vi "AguaClara license agreement.vi"(3 "year":u16) -> (0 "Accepted":bool, 1 "License":string)   [LabVIEW 2015]
panel:
  out "title":string
  in  "OK Button":bool
  in  "I do NOT accept terms of the agreement":bool=TRUE
  in  "I accept terms of the agreement":bool
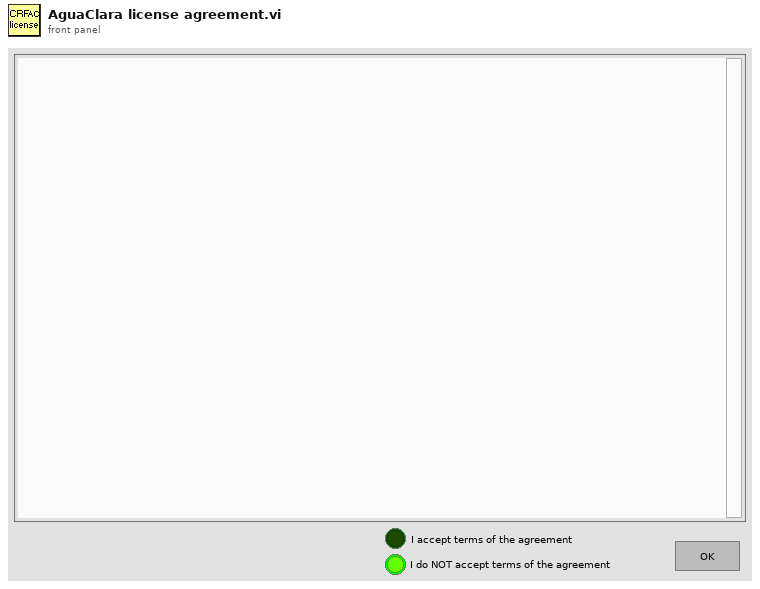
[diagram p1: front panel]
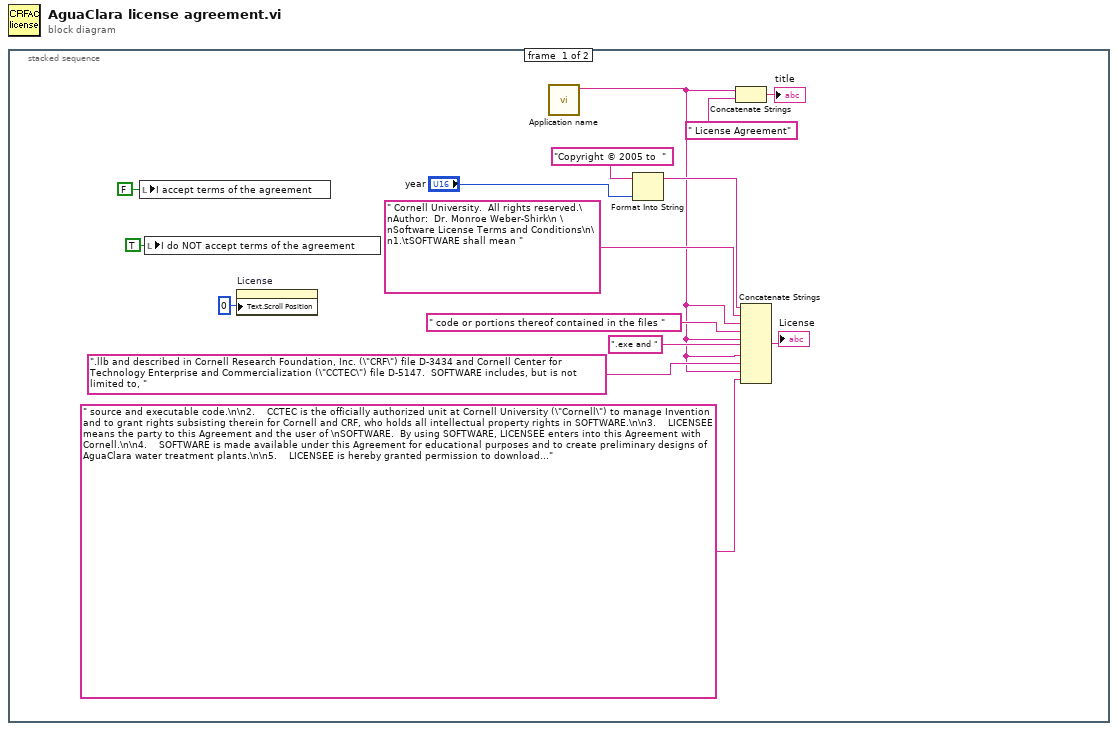
[diagram p0: block diagram]
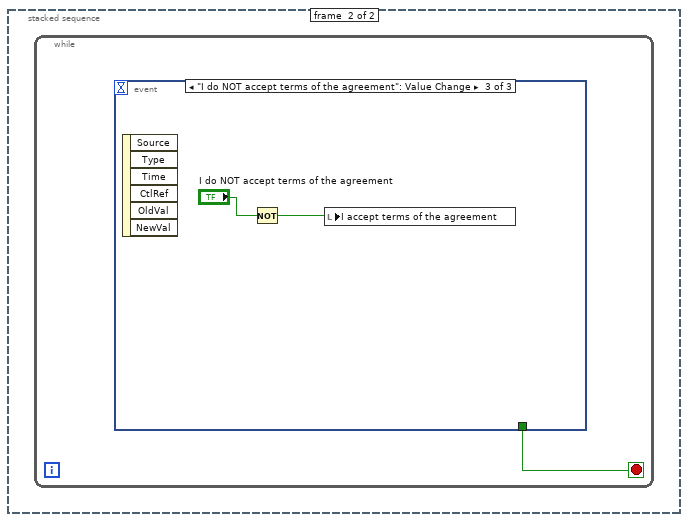
[diagram p2: hidden frame]
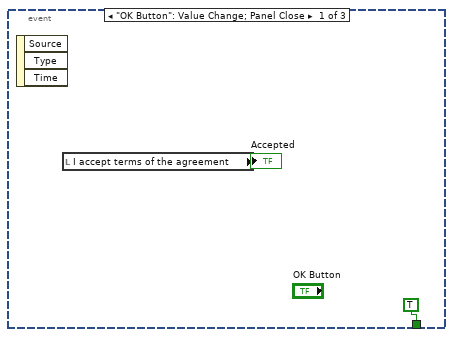
[diagram p3: hidden frame]
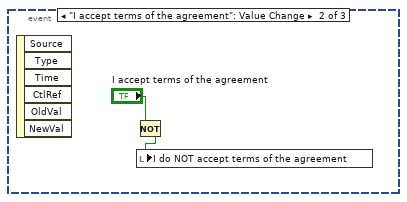
[diagram p4: hidden frame]
diagram:
  n1 = stacked-sequence {
    frame #0 {
      n2 = local write "I accept terms of the agreement"(FALSE ("I accept terms of the agreement")) -> ()
      n3 = local write "I do NOT accept terms of the agreement"(TRUE ("I do NOT accept terms of the agreement")) -> ()
      n4 = property on="License" class="Str"("Text.Scroll Position"=u32 0) -> ()  [unwired: 2 in, 2 out]
      n5 = call "Application name.vi"() -> ("application name"=w1:string)  [unwired: 5 in, 2 out]
      n6 = Format Into String(initial string="Copyright © 2005 to  ", "year") -> (resulting string=w11:string)  [unwired: 2 in, 1 out]
      n7 = Concatenate Strings(w1, " License Agreement" ("string")) -> (→"title":string)
      n8 = Concatenate Strings(w11, " Cornell University.  All rights reserved.\nAuthor:  Dr. Monroe Weber-Shirk\n \nSoftware License Terms and Conditions\n\n1.\tSOFTWARE shall mean ", w1, " code or portions thereof contained in the files ", w1, ".exe and ", w1, ".llb and described in Cornell Research Foundation, Inc. (\"CRF\") file D-3434 and Cornell Center for Technology Enterprise and Commercialization (\"CCTEC\") file D-5147.  SOFTWARE includes, but is not limited to, ", w1, " source and executable code.\n\n2.    CCTEC is the officially authorized unit at Cornell University (\"Cornell\") to manage Invention and to grant rights subsisting therein for Cornell and CRF, who holds all intellectual property rights in SOFTWARE.\n\n3.    LICENSEE means the party to this Agreement and the user of \nSOFTWARE.  By using SOFTWARE, LICENSEE enters into this Agreement with Cornell.\n\n4.    SOFTWARE is made available under this Agreement for educational purposes and to create preliminary designs of AguaClara water treatment plants.\n\n5.    LICENSEE is hereby granted permission to download and execute SOFTWARE provided that this notice accompanies all copies of SOFTWARE.\n\n6.    LICENSEE agrees that the export of SOFTWARE from the United States \nmay require approval from the U.S. government and failure to obtain such approval will result in the immediate termination of this license and may result in criminal liability under U.S. laws.\n\n7.    Cornell provides SOFTWARE on an \"as is\" basis.  Cornell does not warrant, \nguarantee, or make any representations regarding the use or results of SOFTWARE with respect to its correctness, accuracy, reliability or performance.  The entire risk of the use and performance of SOFTWARE is assumed by LICENSEE.  ALL WARRANTIES INCLUDING, WITHOUT LIMITATION, ANY WARRANTY OF FITNESS FOR A PARTICULAR PURPOSE OR MERCHANTABILITY AND ANY WARRANTY OF NONINFRINGEMENT OF PATENTS, COPYRIGHTS, OR ANY OTHER INTELLECTUAL PROPERTY RIGHT ARE HEREBY EXCLUDED.\n\n8.    LICENSEE understands and agrees that neither CCTEC nor Cornell is under any obligation to provide maintenance, support or update services, notices of latent defects, correction of defects, or future versions for SOFTWARE.\n\n9.    Even if advised of the possibility of damages, under no circumstances shall CCTEC or Cornell individually or jointly be liable to LICENSEE or any third party for damages of any character, including, without limitation, direct, indirect, incidental, consequential or special damages, loss of profits, loss of use, loss of goodwill, computer failure or malfunction.  LICENSEE agrees to indemnify and hold harmless CCTEC and Cornell for any and all liability CCTEC or Cornell may incur as a result of use of SOFTWARE by LICENSEE.\n") -> (→"License":string)
    }
    frame #1 {
      n9 = while {
        stop <- w16 stop-if-true
        n10 = event shown="[2] \"I do NOT accept terms of the agreement\": Value Change" {
          selector: _ -> [_ _ _]
          dyn-events: _ -> [_ _ _]
          timeout: _ -> [_ _ _]
          tunnel: [TRUE ("OK Button") _ _] -> w16
          event "OK Button": Value Change; Panel Close {
            n11 = event-data() -> ()  [unwired: 1 in, 3 out]
            n12 = local read "I accept terms of the agreement"() -> (→"Accepted":bool)
          }
          event "I accept terms of the agreement": Value Change {
            n13 = event-data() -> ()  [unwired: 1 in, 6 out]
            n14 = Not(x="I accept terms of the agreement") -> (.not. x?=w19:bool)
            n15 = local write "I do NOT accept terms of the agreement"(w19) -> ()
          }
          event "I do NOT accept terms of the agreement": Value Change {
            n16 = event-data() -> ()  [unwired: 1 in, 6 out]
            n17 = Not(x="I do NOT accept terms of the agreement") -> (.not. x?=w21:bool)
            n18 = local write "I accept terms of the agreement"(w21) -> ()
          }
        }
      }
    }
  }
